vi "_findArgument.vi"(7 "Error If Not Found":bool=TRUE caption="Error If Not Found (T)", 8 "error in (no error)":errorcluster, 10 "Argument":string, 11 "Arguments In":string[](array[string])) -> (0 "error out":errorcluster, 1 "Found":bool, 2 "Value":string, 3 "Arguments Out":string[](array[string]))   [LabVIEW 2013, in "LVAutomationListener.lvlib" / "LVAutomationListener.lvclass"]
doc: "Checks for a given argument and returns its value with whitespace stripped from both the left and right. Can optionally generate an error if the argument is not found. Also reports whether argument was found."
uses:
  LVAutomationListener.lvclass
  _status.ctl
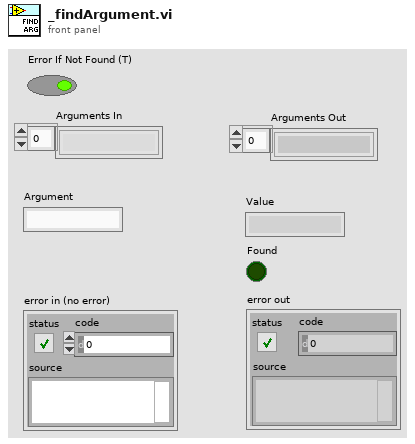
[diagram p1: front panel]
types:
  T1 = typedef "LVAutomationListener.lvlib/LVAutomationListener.lvclass/_status.ctl" = enum16{"Missing Argument", "Unknown Command", "Missing Build Spec Item", "Bad Type", "Compiler Aborted"}
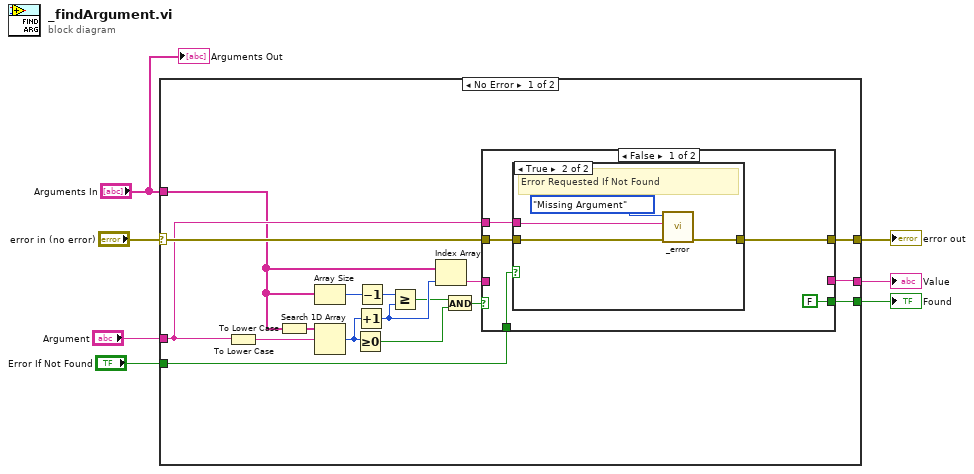
[diagram p0: block diagram]
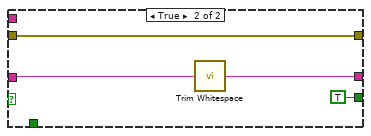
[diagram p3: hidden frame]
diagram:
  n1 = case shown="No Error" "error in (no error)" {
    selector: "error in (no error)" -> [w14 w39]
    tunnel: [w12 w39] -> w6
    tunnel: "Argument" -> [w13 _]
    tunnel: [w10 _] -> w4
    tunnel: [w11 _] -> w3
    tunnel: "Error If Not Found" -> [w9 _]
    tunnel: "Arguments In" -> [w8 _]
    frame No Error {
      n2 = To Lower Case(string=w13) -> (all lower case string=w23:string)
      n3 = To Lower Case(string=w8) -> (all lower case string=w15:string[])
      n4 = Array Size(array=w8) -> (size(s)=w18:i32)
      n5 = Search 1D Array(1D array=w15, element=w23) -> (index of element=w19:i32)  [unwired: 1 in]
      n6 = Greater Or Equal To 0?(x=w19) -> (x >= 0?=w20:bool)
      n7 = Increment(x=w19) -> (x+1=w24:i32)
      n8 = Decrement(x=w18) -> (x-1=w17:i32)
      n9 = Greater Or Equal?(x=w17, y=w24) -> (x >= y?=w16:bool)
      n10 = Index Array(array=w8, index=w24) -> (element=w22:string)
      n11 = And(x=w16, y=w20) -> (x .and. y?=w21:bool)
      n12 = case shown="False" w21 {
        tunnel: w14 -> [w28 w38]
        tunnel: [w27 w38] -> w12
        tunnel: w13 -> [w26 _]
        tunnel: w22 -> [_ w36]
        tunnel: [FALSE TRUE] -> w11
        tunnel: [_ w35] -> w10
        tunnel: w9 -> [w25 _]
        frame False {
          n13 = case shown="True" w25 {
            tunnel: w28 -> [w30 w34]
            tunnel: [w30 w33] -> w27
            tunnel: w26 -> [_ w32]
            frame False {
              # "Don't Error"
            }
            frame True {
              # "Error Requested If Not Found"
              n14 = call "_error.vi"("error in (no error)"=w34, "Additional message"=w32, "Status"=_status."Missing Argument") -> ("error out"=w33:errorcluster)  [unwired: 8 in]
            }
          }
        }
        frame True {
          n15 = call <vilib>:"Trim Whitespace.vi"("string"=w36) -> ("trimmed string"=w35:string)  [unwired: 1 in]
        }
      }
    }
    frame Error {
    }
  }
  "error out" <- w6
  "Value" <- w4
  "Found" <- w3
  "Arguments Out" <- "Arguments In"
